vi "load tags from CSV.vi"(11 "engine configuration in":refnum<class "engine configuration.lvclass">) -> (2 "load attempted":bool, 3 "engine configuration out":refnum<class "engine configuration.lvclass">)   [LabVIEW 2013, in "PL Framework Configuration Tool.lvlib" / "EngineTags.lvclass"]
uses:
  EngineTags.lvclass
  <vilib>/NI/Module Execution Interface/Engine Configuration/engine configuration.lvclass
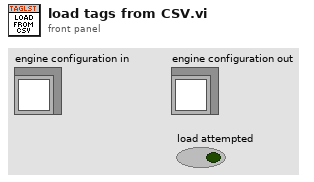
[diagram p1: front panel]
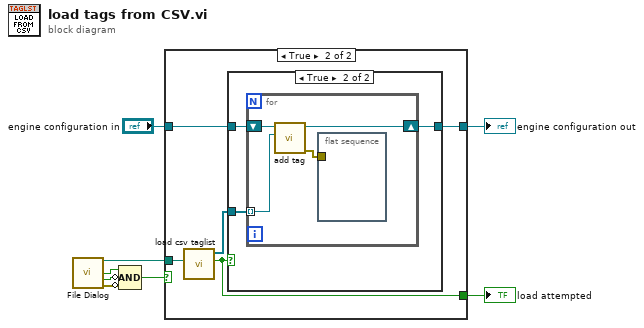
[diagram p0: block diagram]
diagram:
  n1 = call "File Dialog"() -> ("selected path"=w4:path, "exists"=w3:bool, "cancelled"=w2:bool, "error out"=w1:errorcluster)  [unwired: 12 in]
  n2 = Compound Arithmetic op=AND(w3, invert w2, invert w1) -> (w5:bool)
  n3 = case shown="True" w5 {
    tunnel: w4 -> [_ w13]
    tunnel: [_ w12] -> w8
    tunnel: [w9 w10] -> w6
    tunnel: "engine configuration in" -> [w9 w11]
    frame False {
    }
    frame True {
      n4 = call "load csv taglist.vi"("cfg file path"=w13) -> ("ok?"=w12:bool, "tags"=w14:refnum<class "tag descriptor.lvclass">[])  [unwired: 9 in]
      n5 = case shown="True" w12 {
        tunnel: w14 -> [_ w18]
        tunnel: w11 -> [w15 w17]
        tunnel: [w15 w16] -> w10
        frame False {
        }
        frame True {
          n6 = for {
            shift-right: [w22] -> w16
            shift-left: w17 -> [w21]
            tunnel: w18 -> [w20] mode=indexing
            n7 = call <vilib>:"add tag.vi"("tag descriptor"=w20, "engine configuration in"=w21) -> ("error out"=w19:errorcluster, "engine configuration out"=w22:refnum<class "engine configuration.lvclass">)  [unwired: 8 in]
            n8 = flat-sequence {
              tunnel: w19 -> [_]
              frame #0 {
              }
            }
          }
        }
      }
    }
  }
  "load attempted" <- w8
  "engine configuration out" <- w6
